vi "全局1.vi"() -> ()   [LabVIEW 2016, in "数据传输系统.lvlib"]
panel:
  out "读取报文显示":string
  out "发送报文显示":string
  in  "PW":string
  in  "MN":string
  out "QN":string
  out "通讯包字符串":string
  out "数据输出":string
  out "register values":u16[](array[numeric]) caption="读取寄存器的值"
  out "系统编码ST":string="21"
  in  "枚举":enum16{"返回请求应答", "上传数据", "返回执行结果"}(ring)
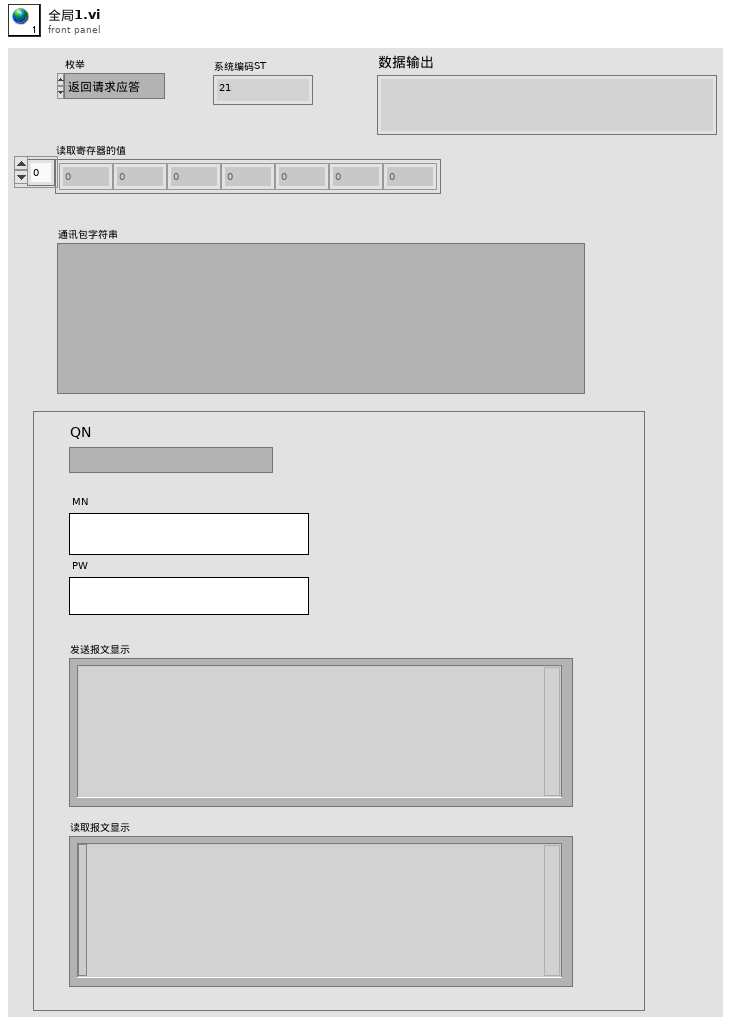
[diagram p1: front panel]
diagram:
